vi "algoritmo_radianos.vi"(3 "AH":dbl, 4 "DEC":dbl, 5 "Latitude Local":dbl) -> (0 "Altura":dbl, 1 "Módulo da Altura":dbl, 2 "Azimute":dbl)   [LabVIEW 2012]
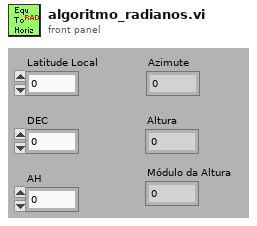
[diagram p1: front panel]
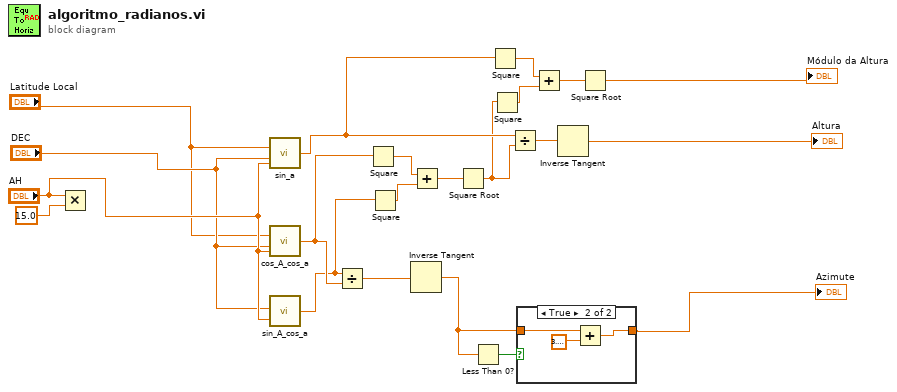
[diagram p0: block diagram]
diagram:
  n1 = Multiply(x="AH", y=15.0) -> ()  [unwired: 1 out]
  n2 = call "sin_a.vi"("AH"="AH", "DEC"="DEC", "Latitude Local"="Latitude Local") -> ("sina"=w11:dbl)
  n3 = call "cos_A_cos_a.vi"("AH"="AH", "DEC"="DEC", "Latitude Local"="Latitude Local") -> ("CosAcosa"=w20:dbl)
  n4 = call "sin_A_cos_a.vi"("AH"="AH", "DEC"="DEC") -> ("sinAcosa"=w19:dbl)
  n5 = Divide(x=w19, y=w20) -> (x/y=w21:dbl)
  n6 = Square(x=w20) -> (x^2=w17:dbl)
  n7 = Square(x=w19) -> (x^2=w16:dbl)
  n8 = Inverse Tangent(1:w21) -> (0:w6:dbl)
  n9 = Add(x=w17, y=w16) -> (x+y=w18:dbl)
  n10 = Square Root(x=w18) -> (sqrt(x)=w10:dbl)
  n11 = Less Than 0?(x=w6) -> (x < 0?=w7:bool)
  n12 = Square(x=w11) -> (x^2=w13:dbl)
  n13 = Square(x=w10) -> (x^2=w14:dbl)
  n14 = Divide(x=w11, y=w10) -> (x/y=w15:dbl)
  n15 = case shown="True" w7 {
    tunnel: w6 -> [w22 w24]
    tunnel: [w22 w25] -> w1
    frame False {
    }
    frame True {
      n16 = Add(x=w24, y=3.141592653589793) -> (x+y=w25:dbl)
    }
  }
  "Azimute" <- w1
  n17 = Add(x=w13, y=w14) -> (x+y=w12:dbl)
  n18 = Inverse Tangent(1:w15) -> (0:→"Altura":dbl)
  n19 = Square Root(x=w12) -> (sqrt(x)=→"Módulo da Altura":dbl)
